vi "NT_GetTopicsList.vi"(11 "String":string) -> (3 "Topic List":T2(array[cluster]) {"NT_Type" items=["NT_Unassigned"=0, "NT_Boolean"=1, "NT_Double"=2, "NT_String"=4, "NT_Raw"=8, "NT_BooleanArray"=16, "NT_DoubleArray"=32, "NT_StringArray"=64, "NT_RPC"=128, "NT_Integer"=256, "NT_Float"=512, "NT_IntegerArray"=1024, "NT_FloatArray"=2048]})   [LabVIEW 2025]
uses:
  <vilib>/Rock Robotics/Network Tables/NT Datatype.ctl
  <vilib>/Rock Robotics/Network Tables/NT Globals.vi
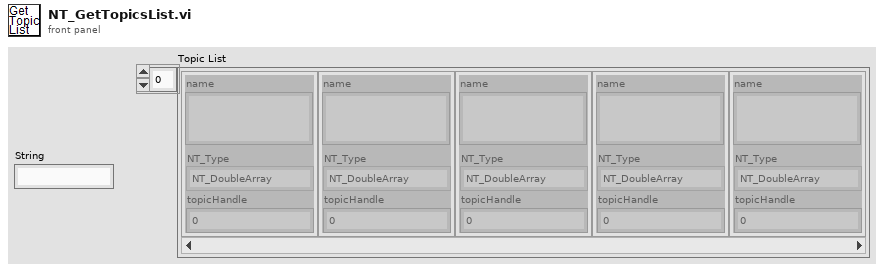
[diagram p1: front panel]
types:
  T1 = typedef "NT Datatype.ctl" = u32
  T2 = cluster{"name":string, "NT_Type":T1, "topicHandle":u32}[]
  T3 = cluster{"name":string, "type":u32, "topic":u32}[]
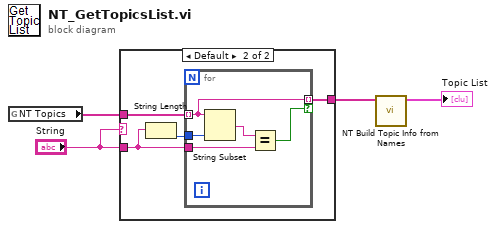
[diagram p0: block diagram]
diagram:
  n1 = global read "NT Globals.vi" "NT Topics"() -> (w2:string[])
  n2 = case shown="Default" "String" {
    tunnel: w2 -> [w5 w9]
    tunnel: "String" -> [_ w8]
    tunnel: [w5 w6] -> w1
    frame "" {
    }
    frame Default {
      n3 = String Length(string=w8) -> (length=w7:i32)
      n4 = for {
        tunnel: w9 -> [w11] mode=indexing
        tunnel: w8 -> [w13]
        tunnel: w7 -> [w14]
        tunnel: [w11] -> w6 mode=indexing if=w10
        n5 = String Subset(string=w11, length (rest)=w14) -> (substring=w12:string)  [unwired: 1 in]
        n6 = Equal?(x=w12, y=w13) -> (x = y?=w10:bool)
      }
    }
  }
  n7 = call <vilib>:"NT Build Topic Info from Names.vi"("NT Topics"=w1) -> ("Topic Info"=→"Topic List":T3)  [unwired: 10 in]
